vi "populate_config_or_settings_combo.vi"(8 "error in (no error)":errorcluster, 9 "type":enum16{"configuration", "settings"}(ring), 10 "combo-box reference":refnum<vi>, 11 "plug-in specification":T1) -> (0 "error out":errorcluster)   [LabVIEW 2017]
uses:
  clusters/plugin_specification.ctl
  <vilib>/regexp/Match Regular Expression.xnode
  xcontrols/XUserDropdown/XUserDropdown/XUserDropdown.xctl
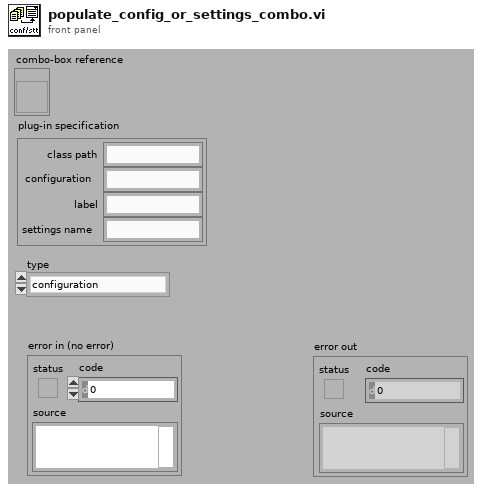
[diagram p1: front panel]
types:
  T1 = typedef "plugin_specification.ctl" = cluster{"class path":string, "configuration":string, "label":string, "settings name":string}
  T2 = typedef "settings_paths_cluster.ctl" = cluster{"base folder":path, "base folder for user":path, "component folder":path, "component file path":path}
  T3 = typedef "configuration_paths_cluster.ctl" = cluster{"base folder":path, "base folder for user":path, "component folder":path, "component file path":path, "main folder":path, "main file":path}
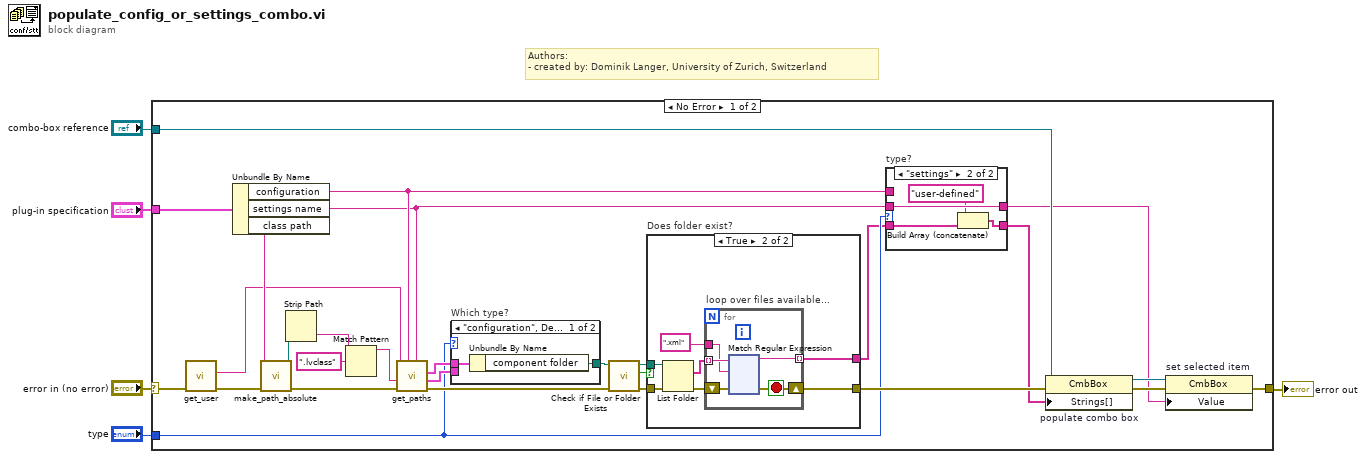
[diagram p0: block diagram]
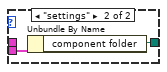
[diagram p4: hidden frame]
diagram:
  # "Authors: \n- created by: Dominik Langer, University of Zurich, Switzerland"
  n1 = case shown="No Error" "error in (no error)" {
    selector: "error in (no error)" -> [w8 w168]
    tunnel: [w15 w168] -> w5
    tunnel: "plug-in specification" -> [w33 _]
    tunnel: "combo-box reference" -> [w18 _]
    tunnel: "type" -> [w14 _]
    frame No Error {
      n2 = call "get_user.vi"("error in (no error)"=w8) -> ("error out"=w7:errorcluster, "username out"=w6:string)  [unwired: 9 in]
      n3 = Unbundle By Name(w33) -> ("configuration"=w13:string, "settings name"=w10:string, "class path"=w28:string)
      n4 = call "make_path_absolute.vi"("error in (no error)"=w7, "relative path"=w28) -> ("error out"=w30:errorcluster, "absolute path"=w29:path)  [unwired: 8 in]
      n5 = Strip Path(path=w29) -> (name=w32:string)  [unwired: 1 out]
      n6 = Match Pattern(string=w32, regular expression=".lvclass") -> (before substring=w25:string)  [unwired: 4 out]
      n7 = call "get_paths.vi"("settings file name (without ending)"=w10, "configuration file name (without ending)"=w13, "error in (no error)"=w30, "component name"=w25, "user"=w6) -> ("error out"=w22:errorcluster, "settings paths"=w26:T2, "configuration paths"=w27:T3)  [unwired: 1 in, 3 out]
      n8 = case "Which type?" shown="\"configuration\", Default" w14 {
        tunnel: w27 -> [w165 _]
        tunnel: [w164 w167] -> w23
        tunnel: w26 -> [_ w166]
        frame "configuration", Default {
          n9 = Unbundle By Name(w165) -> ("component folder"=w164:path)
        }
        frame "settings" {
          n10 = Unbundle By Name(w166) -> ("component folder"=w167:path)
        }
      }
      n11 = call <vilib>:"Check if File or Folder Exists.vi"("error in (no error)"=w22, "path"=w23) -> ("error out"=w21:errorcluster, "file or folder exists?"=w20:bool, "dup path"=w24:path)  [unwired: 7 in]
      n12 = case "Does folder exist?" shown="True" w20 {
        tunnel: [w40 w42] -> w16
        tunnel: w24 -> [_ w44]
        tunnel: w21 -> [w40 w43]
        tunnel: [_ w41] -> w12
        frame False {
        }
        frame True {
          n13 = List Folder(path=w44, error in=w43) -> (filenames=w45:string[], error out=w46:errorcluster)  [unwired: 4 out]
          n14 = for "loop over files available..." {
            tunnel: w45 -> [w52] mode=indexing
            tunnel: [w51] -> w41 mode=indexing
            tunnel: ".xml" ("regular expression") -> [w49]
            shift-right: [w48] -> w42
            shift-left: w46 -> [w50]
            stop <- w48 stop-if-true
            n15 = xnode "Match Regular Expression"("input string"=w52, "regular expression"=w49, "error in"=w50) -> ("before match"=w51:string, "error out"=w48:errorcluster)  [unwired: 1 in, 5 out]
          }
        }
      }
      n16 = case "type?" shown="\"settings\"" w14 {
        tunnel: w10 -> [_ w39]
        tunnel: w13 -> [w35 _]
        tunnel: [w35 w39] -> w9
        tunnel: w12 -> [w34 w38]
        tunnel: [w34 w37] -> w11
        frame "configuration", Default {
        }
        frame "settings" {
          n17 = Build Array (concatenate)("user-defined" ("before match"), w38) -> (w37:string[])
        }
      }
      n18 = property on="populate combo box" class="CmbBox"(reference=w18, error in=w16, "Strings[]"=w11) -> (reference out=w17:refnum<vi>, error out=w19:errorcluster)
      n19 = property on="set selected item" class="CmbBox"(reference=w17, error in=w19, "Value"=w9) -> (error out=w15:errorcluster)  [unwired: 1 out]
    }
    frame Error {
    }
  }
  "error out" <- w5
